vi "1.8.0 Mutation.vi"(8 "error in":errorcluster, 11 "Device Ref in":T1 format="%.0x") -> (0 "error out":errorcluster, 3 "Device Ref out":T1 format="%.0x")   [LabVIEW 2015, in "AIT 429 System Explorer.lvlib"]
uses:
  AIT 429 System Explorer.lvlib
  <vilib>/NI Veristand/Custom Device API/Custom Device Item Ref.ctl
  NationalInstruments.VeriStand.SystemStorage
  Shared/Controls and Global/Global.vi
  <vilib>/NI Veristand/Custom Device Tools/Custom Device Utility Library/NI VeriStand - Search for Item by Name.vi
  <vilib>/NI VeriStand/Custom Device Tools/Custom Device Utility Library/Custom Device Utility Library.lvlib
  Shared/ARINC 429 Shared.lvlib
  <vilib>/NI VeriStand/Custom Device API/Custom Device API.lvlib
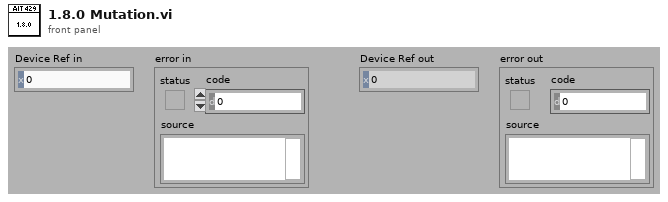
[diagram p1: front panel]
types:
  T1 = typedef "Custom Device API.lvlib/Custom Device Item Ref.ctl" = u64
  T2 = typedef "Custom Device API.lvlib/Custom Device Pointer.ctl" = refnum<k24>
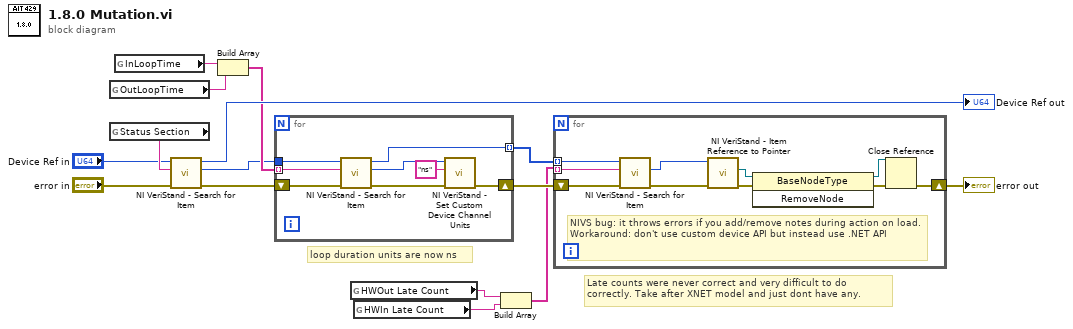
[diagram p0: block diagram]
diagram:
  # "Late counts were never correct and very difficult to do correctly. Take after XNET model and just dont have any."
  # "loop duration units are now ns"
  n1 = global read "Global.vi" "OutLoopTime"() -> (w13:string)
  n2 = global read "Global.vi" "Status Section"() -> (w9:string)
  n3 = global read "Global.vi" "InLoopTime"() -> (w12:string)
  n4 = call-poly <vilib>:"NI VeriStand - Search for Item.vi"("error in"="error in", "Item Name"=w9, "Section Ref in"="Device Ref in") -> ("error out"=w11:errorcluster, "Item Ref"=w10:T1, "Section Ref out"=→"Device Ref out":T1)  [unwired: 5 in, 1 out]
  n5 = Build Array(w12, w13) -> (w14:string[])
  n6 = for {
    tunnel: w10 -> [w23]
    shift-right: [w19] -> w5
    shift-left: w11 -> [w22]
    tunnel: w14 -> [w21] mode=indexing
    tunnel: [w16] -> w6 mode=indexing
    n7 = call-poly <vilib>:"NI VeriStand - Search for Item.vi"("error in"=w22, "Item Name"=w21, "Section Ref in"=w23) -> ("error out"=w20:errorcluster, "Item Ref"=w18:T1, "Section Ref out"=w16:T1)  [unwired: 5 in, 1 out]
    n8 = call <vilib>:"NI VeriStand - Set Custom Device Channel Units.vi"("error in (no error)"=w20, "Units"="ns", "Channel Ref in"=w18) -> ("error out"=w19:errorcluster)  [unwired: 7 in, 1 out]
  }
  n9 = global read "Global.vi" "HWOut Late Count"() -> (w4:string)
  n10 = global read "Global.vi" "HWIn Late Count"() -> (w3:string)
  n11 = Build Array(w4, w3) -> (w2:string[])
  n12 = for {
    tunnel: w6 -> [w33] mode=indexing
    shift-right: [w25] -> w1
    shift-left: w5 -> [w32]
    tunnel: w2 -> [w31] mode=indexing
    # "NIVS bug: it throws errors if you add/remove notes during action on load. Workaround: don't use custom device API but instead use .NET API"
    n13 = call-poly <vilib>:"NI VeriStand - Search for Item.vi"("error in"=w32, "Item Name"=w31, "Section Ref in"=w33) -> ("error out"=w30:errorcluster, "Item Ref"=w29:T1)  [unwired: 5 in, 2 out]
    n14 = call <vilib>:"NI VeriStand - Item Reference to Pointer.vi"("error in (no error)"=w30, "Item Ref in"=w29) -> ("error out"=w27:errorcluster, "Node Pointer"=w28:T2)  [unwired: 6 in, 2 out]
    n15 = invoke class="BaseNodeType" method="RemoveNode"(reference=w28, error in=w27) -> (reference out=w24:T2, error out=w26:errorcluster)  [unwired: 1 in, 1 out]
    n16 = Close Reference(reference=w24, error in (no error)=w26) -> (error out=w25:errorcluster)
  }
  "error out" <- w1
